vi "Add Cashier.vi"(8 "error in (no error)":errorcluster, 11 "Coffee Shop in":refnum<class "Coffee Shop.lvclass">) -> (0 "error out":errorcluster, 3 "Coffee Shop out":refnum<class "Coffee Shop.lvclass">)   [LabVIEW 2023, in "Coffee Shop.lvlib" / "Coffee Shop.lvclass"]
doc: "Add a new cashier actor to the coffee shop"
uses:
  Coffee Shop.lvclass
  c:/dev/_r/4/eng/lv-core/lvpostprocessingd/lv_mc_x86_64/dist_i386/vi.lib/ActorFramework/Actor/Actor.lvclass
  Worker/Cashier/Cashier.lvclass
  Entity Table/Entity Data.ctl
  Entity Types.ctl
  Coffee Shop.lvclass/Coffee Shop.ctl
  Entity Table/Entity Table.lvclass
  <vilib>/ActorFramework/Actor/Actor.lvclass
panel:
  in  "Waiting":string="Waiting..."
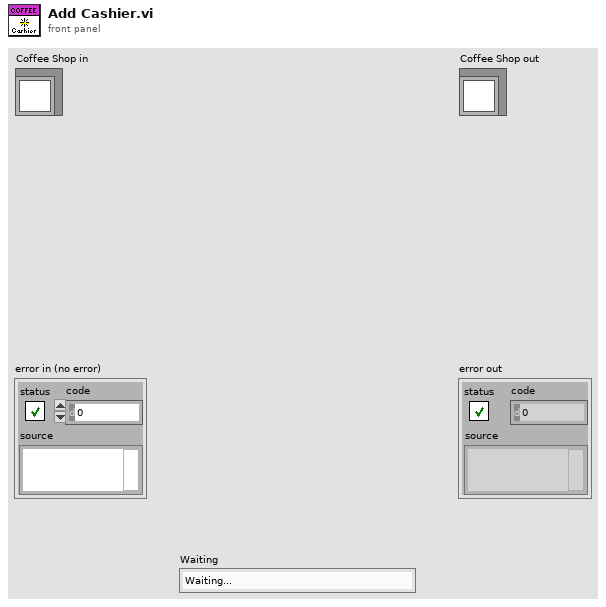
[diagram p1: front panel]
types:
  T1 = typedef "Coffee Shop.lvlib/Coffee Shop.lvclass/Entity Types.ctl" = enum16{"Customer", "Cashier", "Barista"}
  T2 = typedef "Entity Table.lvclass/Entity Data.ctl" = cluster{"Name":string, "Status":string}
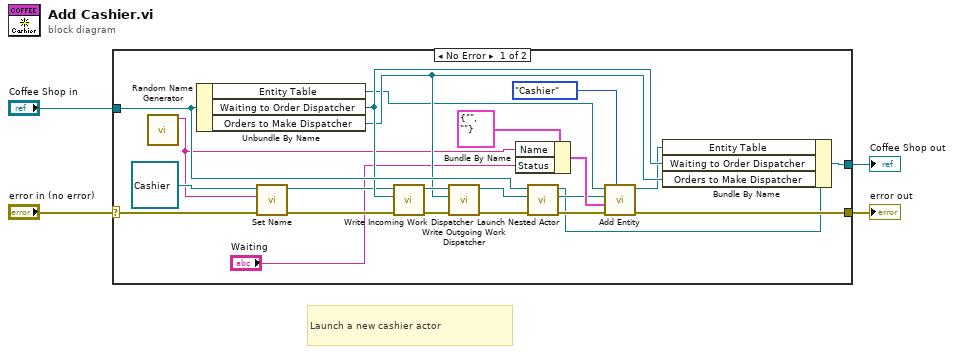
[diagram p0: block diagram]
diagram:
  # "Launch a new cashier actor"
  n1 = case shown="No Error" "error in (no error)" {
    selector: "error in (no error)" -> [w25 w29]
    tunnel: [w26 w29] -> w3
    tunnel: [w27 w28] -> w1
    tunnel: "Coffee Shop in" -> [w24 w28]
    frame No Error {
      n2 = call "Random Name Generator.vi"() -> ("Name"=w14:string)  [unwired: 11 in]
      n3 = Unbundle By Name(w24) -> ("Entity Table"=w8:refnum<class "Entity Table.lvclass">, "Waiting to Order Dispatcher"=w20:refnum<class "Message Enqueuer.lvclass">, "Orders to Make Dispatcher"=w19:refnum<class "Message Enqueuer.lvclass">)
      n4 = call-dynamic "Set Name.vi"("error in (no error)"=w25, "Name"=w14, "Person in"=refnum<class "Cashier.lvclass"> refnum ("Cashier.lvclass")) -> ("error out"=w17:errorcluster, "Person out"=w16:refnum<class "Cashier.lvclass">)  [unwired: 7 in]
      n5 = call-dynamic "Write Incoming Work Dispatcher.vi"("error in (no error)"=w17, "Incoming Work Dispatcher Queue"=w20, "Worker in"=w16) -> ("error out"=w22:errorcluster, "Worker out"=w23:refnum<class "Cashier.lvclass">)  [unwired: 7 in]
      n6 = call-dynamic "Write Outgoing Work Dispatcher.vi"("error in (no error)"=w22, "Outgoing Work Dispatcher Queue"=w19, "Worker in"=w23) -> ("error out"=w21:errorcluster, "Worker out"=w6:refnum<class "Cashier.lvclass">)  [unwired: 7 in]
      n7 = Bundle By Name(cluster=T2 {"Name"="", "Status"=""} ("Entity"), "Name"=w14, "Status"="Waiting") -> (w11:T2)
      n8 = call <vilib>:"Launch Nested Actor.vi"("error in (no error)"=w21, "Nested Actor"=w6, "Caller Actor in"=w24) -> ("error out"=w10:errorcluster, "Nested Actor's Enqueuer"=w9:refnum<class "Message Enqueuer.lvclass">, "Caller Actor out"=w5:refnum<class "Coffee Shop.lvclass">)  [unwired: 6 in]
      n9 = call "Add Entity.vi"("entity type"=Entity_Types."Cashier", "error in (no error)"=w10, "entity details"=w11, "enqueuer"=w9, "Entity Table in"=w8) -> ("error out"=w26:errorcluster, "Entity Table out"=w7:refnum<class "Entity Table.lvclass">)  [unwired: 5 in]
      n10 = Bundle By Name(cluster=w5, "Entity Table"=w7, "Waiting to Order Dispatcher"=w20, "Orders to Make Dispatcher"=w19) -> (w27:refnum<class "Coffee Shop.lvclass">)
    }
    frame Error {
    }
  }
  "error out" <- w3
  "Coffee Shop out" <- w1
